vi "EDIT SALE DESCRIPTION.vi"(11 "REFERENCES":T1) -> ()   [LabVIEW 2019]
uses:
  Controls/References Cluster.ctl
  <vilib>/userDefined/High Color/IMAQdx.ctl
  Controls/Custom Calendar/Custom Calendar.xctl
  <vilib>/addons/database/Connection.llb/DB Tools Open Connec (String).vi
  <vilib>/addons/database/Connection.llb/Conn Execute.vi
  <vilib>/addons/database/Recordset.llb/Rec Destroy - Connection.vi
  <vilib>/addons/database/NI_Database_API.lvlib
types:
  T1 = typedef "References Cluster.ctl" = cluster{"MAIN PAGES":refnum<vi>, "ADD/EDIT ITEM REFERENCES":cluster{"Identifier":refnum<vi>, "BYU ICN #":refnum<vi>, "Item Description":refnum<vi>, "Comments":refnum<vi>, "Checked Out Date":refnum<vi>, "Due Date":refnum<vi>, "Check Out Location":refnum<vi>, "Reminder Count":refnum<vi>, "Most Recent Reminder Date":refnum<vi>, "BYU ID #":refnum<vi>, "Building/Room":refnum<vi>, "Location in Room":refnum<vi>, "Manual":refnum<vi>, "Manufacturer":refnum<vi>, "Model #":refnum<vi>, "Serial #":refnum<vi>, "Date Acquired":refnum<vi>, "ADD/EDIT ITEM LABEL":refnum<vi>, "ARCHIVE ITEM":refnum<vi>, "Archive Item Inputs":refnum<vi>, "Reminder Notes":refnum<vi>, "DUPLICATE ITEM":refnum<vi>}, "ADD/EDIT USER REFERENCES":cluster{"BYU ID # (##-###-####)":refnum<vi>, "First Name":refnum<vi>, "Last Name":refnum<vi>, "Phone Number (###-###-####)":refnum<vi>, "Email":refnum<vi>, "Department":refnum<vi>, "Graduation Status":refnum<vi>, "Anticipated Graduation Year":refnum<vi>, "Credit Score":refnum<vi>, "Date Added":refnum<vi>, "Graduation Clearance Date":refnum<vi>, "Picture File Name":refnum<vi>, "ADD/EDIT USER LABEL":refnum<vi>, "Department Map":refnum<vi>, "Status Map":refnum<vi>, "Anticipated Graduation Year Map":refnum<vi>, "User Agreement":refnum<vi>, "User Comments":refnum<vi>, "Camera":refnum<vi>}, "RETURN ITEM REFERENCES":cluster{"Item or Person:":refnum<vi>, "Search Return Results":refnum<vi>, "What are you searching for?":refnum<vi>}, "SEARCH DATABASE REFERENCES":cluster{"What to Search For:":refnum<vi>, "Where to Search":refnum<vi>, "Column to Search In":refnum<vi>, "Column to Sort By":refnum<vi>, "Search Database Results":refnum<vi>, "Inventory Column Selector":refnum<vi>, "User Column Selector":refnum<vi>, "Inventory Archive Column Selector":refnum<vi>, "User Archive Column Selector":refnum<vi>, "Sales Tracking Column Selector":refnum<vi>, "Checked In Archive Column Selector":refnum<vi>, "Restore User":refnum<vi>, "Date Range":refnum<vi>, "Dates Less Than":refnum<vi>, "Dates Greater Than":refnum<vi>, "Search Print Receipt":refnum<vi>, "Edit Sale Description":refnum<vi>}, "USER ITEMS REFERENCES":cluster{"USER'S INFORMATION":refnum<vi>, "User's Checked Out Items":refnum<vi>, "User Info Comments":refnum<vi>, "SEE USER INFO COMMENTS":refnum<vi>}, "EDIT ITEMS REFERENCES":cluster{"New Check Out Location":refnum<vi>, "Items to Edit":refnum<vi>, "Edit Items Due Date":refnum<vi>, "New Reminder Notes":refnum<vi>, "New Item Description":refnum<vi>}, "CHECK OUT ITEMS REFERENCES":cluster{"Enter Item:":refnum<vi>, "Check Out Items Due Date":refnum<vi>, "Check Out Location":refnum<vi>, "Items to be Checked Out":refnum<vi>, "Possible Items":refnum<vi>, "Altered Item Description":refnum<vi>}, "TRANSFER ITEMS REFERENCES":cluster{"Search Parameter":refnum<vi>, "What to Match":refnum<vi>, "Matching Individuals":refnum<vi>, "Items to be Transferred":refnum<vi>}, "SETTINGS REFERENCES":cluster{"PSC Database Settings":refnum<vi>, "PSC Sales Item Spreadsheet":refnum<vi>}, "PSC SALES REFERENCES":cluster{"BYU ID CARD #":refnum<vi>, "Sale Description":refnum<vi>, "Scan or Enter Item Name":refnum<vi>, "Items to be Sold":refnum<vi>, "Grand Total":refnum<vi>, "Item List":refnum<vi>}}
  T2 = cluster{"What to Search For:":refnum<vi>, "Where to Search":refnum<vi>, "Column to Search In":refnum<vi>, "Column to Sort By":refnum<vi>, "Search Database Results":refnum<vi>, "Inventory Column Selector":refnum<vi>, "User Column Selector":refnum<vi>, "Inventory Archive Column Selector":refnum<vi>, "User Archive Column Selector":refnum<vi>, "Sales Tracking Column Selector":refnum<vi>, "Checked In Archive Column Selector":refnum<vi>, "Restore User":refnum<vi>, "Date Range":refnum<vi>, "Dates Less Than":refnum<vi>, "Dates Greater Than":refnum<vi>, "Search Print Receipt":refnum<vi>, "Edit Sale Description":refnum<vi>}
  T3 = typedef "NI_Database_API.lvlib/Conn ObjectReference.ctl" = refnum<k1>
  T4 = typedef "NI_Database_API.lvlib/Rec ObjectReference.ctl" = refnum<k1>
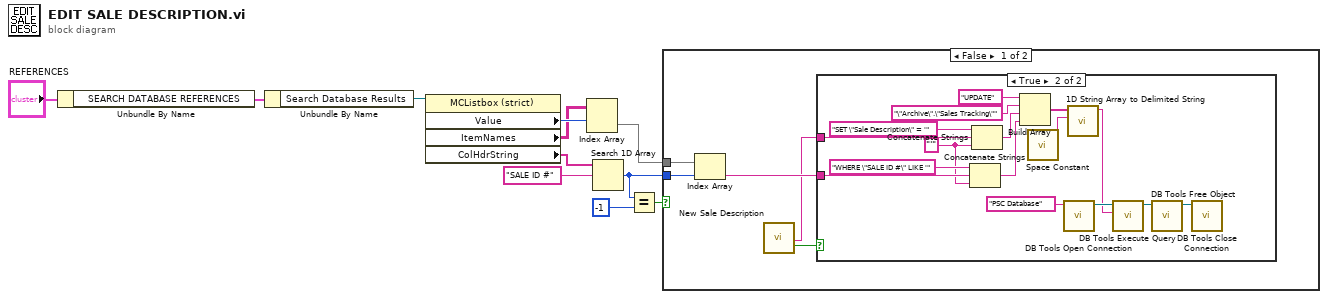
[diagram p0: block diagram]
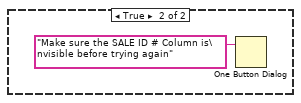
[diagram p3: hidden frame]
diagram:
  n1 = Unbundle By Name("REFERENCES") -> ("SEARCH DATABASE REFERENCES"=w10:T2)
  n2 = Unbundle By Name(w10) -> ("Search Database Results"=w9:refnum<vi>)
  n3 = property class="MCListbox (strict)"(reference=w9) -> ("Value"=w8:i32, "ItemNames"=w7:string[][], "ColHdrString"=w5:string[])  [unwired: 1 in, 2 out]
  n4 = Index Array(array=w7, index (row)=w8) -> (element=w6:string[])  [unwired: 1 in]
  n5 = Search 1D Array(1D array=w5, element="SALE ID #") -> (index of element=w2:i32)  [unwired: 1 in]
  n6 = Equal?(x=w2, y=-1) -> (x = y?=w1:bool)
  n7 = case shown="False" w1 {
    tunnel: w6 -> [w16 _]
    tunnel: w2 -> [w15 _]
    frame False {
      n8 = Index Array(array=w16, index=w15) -> (element=w13:string)
      n9 = call "New Sale Description"() -> ("New Sale Description"=w12:string, "OK"=w14:bool)  [unwired: 17 in, 1 out]
      n10 = case shown="True" w14 {
        tunnel: w13 -> [_ w24]
        tunnel: w12 -> [_ w26]
        frame False {
        }
        frame True {
          w23 = "'" ("string")
          n11 = Concatenate Strings("WHERE \"SALE ID #\" LIKE '" ("string"), w24, w23) -> (w22:string)
          n12 = Concatenate Strings("SET \"Sale Description\" = '" ("string"), w26, w23) -> (w32:string)
          n13 = Build Array("UPDATE" ("string"), "\"Archive\".\"Sales Tracking\"" ("table"), w32, w22) -> (w31:string[])
          n14 = call <vilib>:"Space Constant.vi"() -> ("String"=w30:string)
          n15 = call-poly <vilib>:"DB Tools Open Connection.vi"("connection information"="PSC Database" ("table")) -> ("connection reference"=w21:T3)  [unwired: 7 in, 1 out]
          n16 = call <vilib>:"1D String Array to Delimited String.vi"("delimiter"=w30, "string array"=w31) -> ("delimited string"=w18:string)  [unwired: 9 in]
          n17 = call-poly <vilib>:"DB Tools Execute Query.vi"("SQL query"=w18, "connection reference"=w21) -> ("recordset reference"=w20:T4)  [unwired: 6 in, 1 out]
          n18 = call-poly <vilib>:"DB Tools Free Object.vi"("recordset reference"=w20) -> ("connection reference"=w17:T3)  [unwired: 9 in, 1 out]
          n19 = call <vilib>:"DB Tools Close Connection.vi"("connection reference"=w17) -> ()  [unwired: 6 in, 1 out]
        }
      }
    }
    frame True {
      n20 = One Button Dialog(message="Make sure the SALE ID # Column is\nvisible before trying again") -> ()  [unwired: 1 in, 1 out]
    }
  }
